vi "Read Exporter Name.vi"(11 "CDependencyInspection in":refnum<class "CDependencyInspection.lvclass">) -> (2 "Name":string, 3 "CDependencyInspection out":refnum<class "CDependencyInspection.lvclass">)   [LabVIEW 2020, in "DependencyInspection.lvlib" / "CDependencyInspection.lvclass"]
uses:
  CDependencyInspection.lvclass
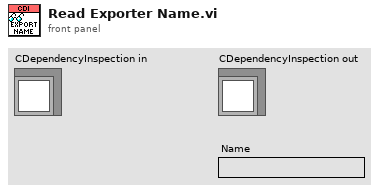
[diagram p1: front panel]
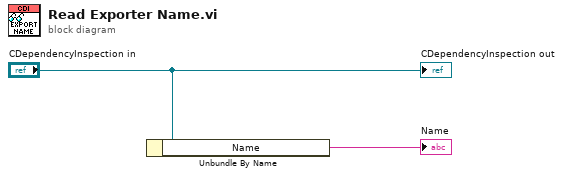
[diagram p0: block diagram]
diagram:
  n1 = Unbundle By Name("CDependencyInspection in") -> ("Name"=→"Name":string)
  "CDependencyInspection out" <- "CDependencyInspection in"
